vi "format_time.vi"(1 "Frame Time Stamp":timestamp=timestamp(3252424354.9818 s since 1904-01-01) format="%<%.4X\n%x>T") -> (0 "output string":string="Frame time stamp: \tJanuary 23 2007: 12:12:34:.9818\r\n")   [LabVIEW 2014]
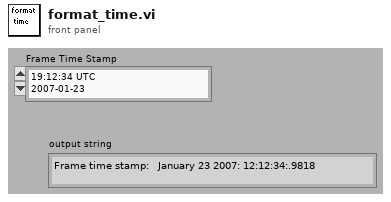
[diagram p1: front panel]
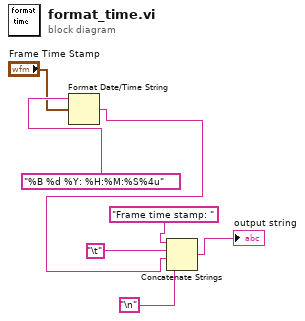
[diagram p0: block diagram]
diagram:
  n1 = Format Date/Time String(time format string (%c)="%B %d %Y: %H:%M:%S%4u", seconds (now)="Frame Time Stamp") -> (date/time string=w3:string)  [unwired: 1 in]
  n2 = Concatenate Strings("Frame time stamp: ", "\t", w3, "\n") -> (→"output string":string)
